vi "5ship.vi"(0 "Array":u16[][](array[ring])) -> (2 "Array 2":u16[][](array[ring]))   [LabVIEW 2014]
panel:
  out "Boolean":bool
  in  "Array 5":u16[][](array[ring])=[[1, 1, 1, 1, 1]]
  in  "Array 3":u16[][](array[ring])=[[1], [1], [1], [1], [1]]
  in  "Raw":i32=1
  in  "Column":i32=1
  in  "?":bool
  in  "?":enum16{"horizon", "vertical"}(ring)
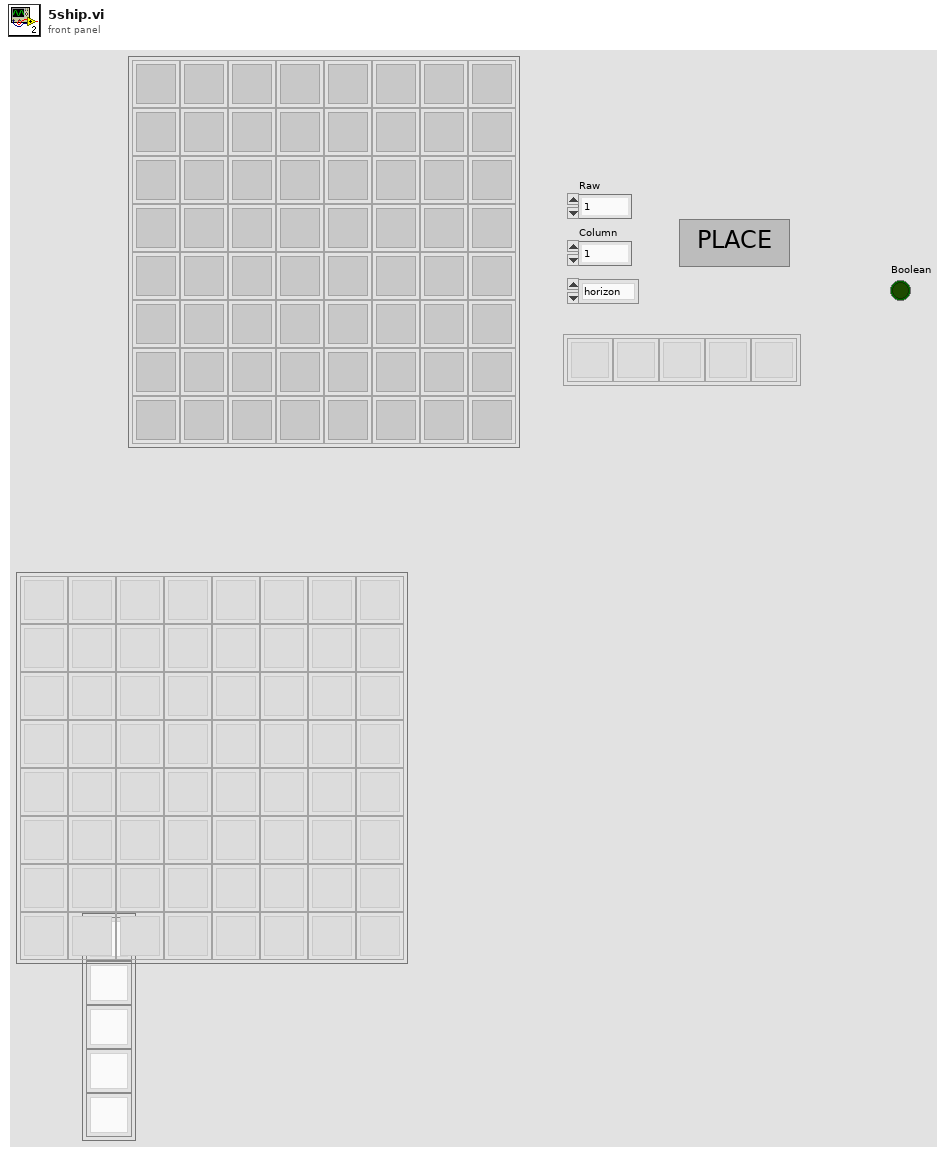
[diagram p1: front panel]
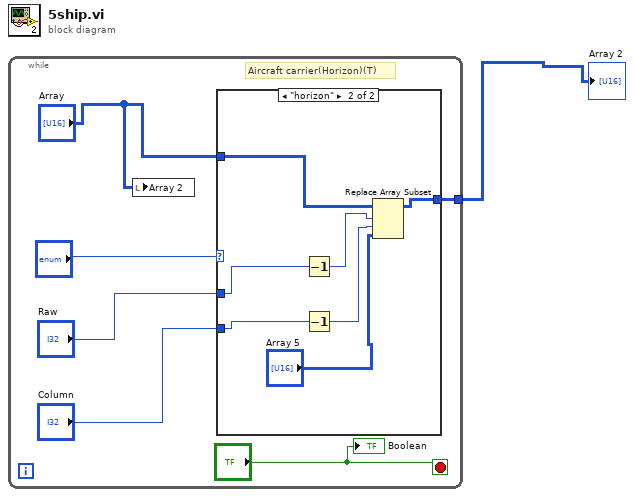
[diagram p0: block diagram]
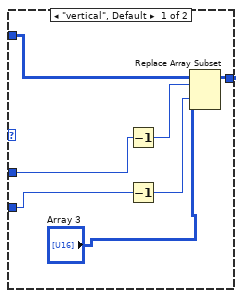
[diagram p2: hidden frame]
diagram:
  n1 = while {
    tunnel: [w7] -> w1
    stop <- "?" stop-if-true
    # "Aircraft carrier(Horizon)(T)"
    n2 = local write "Array 2"("Array") -> ()
    n3 = case shown="\"horizon\"" "?" {
      tunnel: [w11 w18] -> w7
      tunnel: "Raw" -> [w10 w17]
      tunnel: "Column" -> [w9 w16]
      tunnel: "Array" -> [w8 w15]
      frame "vertical", Default {
        n4 = Decrement(x=w10) -> (x-1=w14:i32)
        n5 = Decrement(x=w9) -> (x-1=w13:i32)
        n6 = Replace Array Subset(array=w8, new element="Array 3", index (row)=w14, index (col)=w13) -> (w11:u16[][])
      }
      frame "horizon" {
        n7 = Decrement(x=w17) -> (x-1=w20:i32)
        n8 = Decrement(x=w16) -> (x-1=w19:i32)
        n9 = Replace Array Subset(array=w15, new element="Array 5", index (row)=w20, index (col)=w19) -> (w18:u16[][])
      }
    }
    "Boolean" <- "?"
  }
  "Array 2" <- w1
